vi "readLSdata.vi"(8 "error in (no error)":errorcluster, 10 "LS Loop AI":fxp<+/-,25,5>[](array[numeric])=[0.0, 0.0, 0.0, 0.0, 0.0, 0.0, 0.0, 0.0, 0.0], 11 "PositionMeas in":refnum<class "PositionMeas.lvclass">) -> (0 "error out":errorcluster, 3 "PositionMeas out":refnum<class "PositionMeas.lvclass">)   [LabVIEW 2020]
doc: "Update data from the Low-Speed AI loop and store it in the PositionMeas data storage"
uses:
  PositionMeas.lvclass
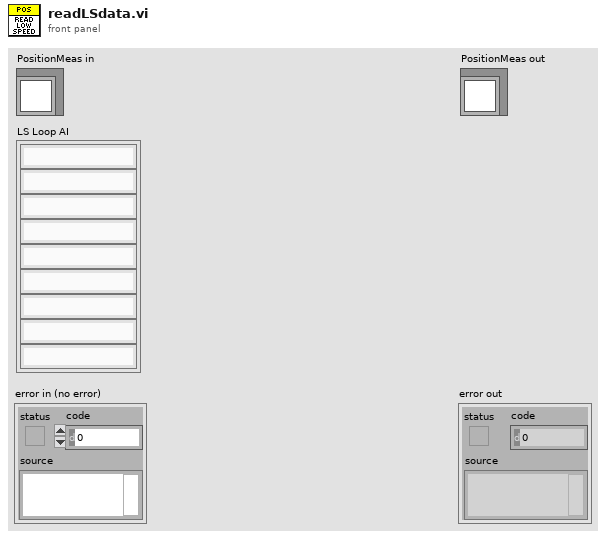
[diagram p1: front panel]
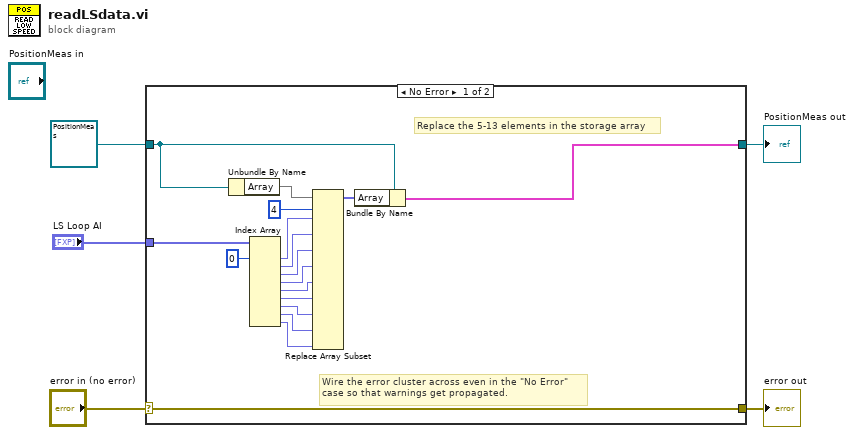
[diagram p0: block diagram]
diagram:
  n1 = case shown="No Error" "error in (no error)" {
    selector: "error in (no error)" -> [w22 w24]
    tunnel: [w22 w24] -> w4
    tunnel: [w12 w23] -> w3
    tunnel: refnum<class "PositionMeas.lvclass"> refnum ("PositionMeas.lvclass") -> [w20 w23]
    tunnel: "LS Loop AI" -> [w18 _]
    frame No Error {
      # "Replace the 5-13 elements in the storage array"
      # "Wire the error cluster across even in the \"No Error\"\ncase so that warnings get propagated."
      n2 = Unbundle By Name(w20) -> ("Array"=w21)
      n3 = Index Array(array=w18, index #1=0 ("index")) -> (element #1=w17:fxp<+/-,25,5>, element #2=w16:fxp<+/-,25,5>, element #3=w15:fxp<+/-,25,5>, element #4=w14:fxp<+/-,25,5>, element #5=w11:fxp<+/-,25,5>, element #6=w9:fxp<+/-,25,5>, element #7=w8:fxp<+/-,25,5>, element #8=w7:fxp<+/-,25,5>, element #9=w6:fxp<+/-,25,5>)  [unwired: 8 in]
      n4 = Replace Array Subset(array=w21, new element #1=w17, index #1=4 ("index"), new element #2=w16, new element #3=w15, new element #4=w14, new element #5=w11, new element #6=w9, new element #7=w8, new element #8=w7, new element #9=w6) -> (w13:fxp<+/-,25,5>[])  [unwired: 8 in]
      n5 = Bundle By Name(cluster=w20, "Array"=w13) -> (w12:cluster{})
    }
    frame Error {
    }
  }
  "error out" <- w4
  "PositionMeas out" <- w3
